vi "ShieldOnly.vi"() -> ()   [LabVIEW 2014]
panel:
  in  "stop":bool
  out "Position in Inches":ext format="%.4f"
  out "Readout":string
  in  "Steps":string(combo)
  in  "Power":bool
  in  "Abort":bool
  in  "Home":bool
  in  "Move":bool
  # "When Readout reads \"\\FF/0'0\\00\\03\\r\\n\", the motor is ready to be used."
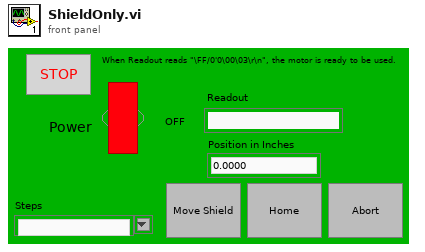
[diagram p1: front panel]
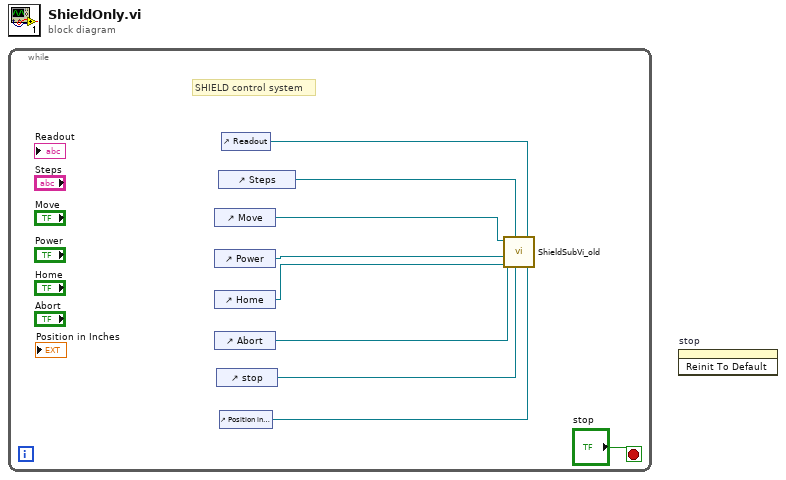
[diagram p0: block diagram]
diagram:
  n1 = while {
    stop <- "stop" stop-if-true
    # "SHIELD control system"
    n2 = control-ref of="Move"() -> (w9:refnum<vi>)
    n3 = control-ref of="Power"() -> (w5:refnum<vi>)
    n4 = control-ref of="Home"() -> (w3:refnum<vi>)
    n5 = control-ref of="Abort"() -> (w8:refnum<vi>)
    n6 = control-ref of="stop"() -> (w1:refnum<vi>)
    n7 = control-ref of="Steps"() -> (w6:refnum<vi>)
    n8 = control-ref of="Position in Inches"() -> (w7:refnum<vi>)
    n9 = control-ref of="Readout"() -> (w4:refnum<vi>)
    n10 = call "ShieldSubVi_old.vi"("DigNum Refnum"=w7, "Str Refnum (Pos readout)"=w4, "Bool Refnum (stop)"=w1, "CmbBox Refnum"=w6, "Bool Refnum (home)"=w3, "Bool Refnum (power)"=w5, "Bool Refnum (abort)"=w8, "Bool Refnum (move)"=w9) -> ()
  }
  n11 = invoke on="stop" class="Bool (strict)" method="Reinit To Default"() -> ()  [unwired: 3 in, 3 out]
